vi "test6-Interrupt_Queue.vi"(8 "error in (no error)":errorcluster, 11 "TestCase in":refnum<class "testcase-CSMGlobalLog.lvclass">) -> (0 "error out":errorcluster, 3 "TestCase out":refnum<class "testcase-CSMGlobalLog.lvclass">)   [LabVIEW 2017, in "testcase-CSMGlobalLog.lvclass"]
uses:
  testcase-CSMGlobalLog.lvclass
  testcase-CSMGlobalLog.lvclass/testcase-CSMGlobalLog.ctl
  05ebe40f-4c18-45b8-8385-0deae4bc461c.vi
  74c550d6-8d72-4fbc-9b84-854ca9ba218d.vi
  f2908a69-50b3-4358-8c93-3e573ca7d2ca.vi
  <vilib>/addons/_JKI Toolkits/VI Tester/TestCase.llb/TestCase.lvclass
  src/user.lib/_NEVSTOP/Communicable State Machine(CSM)/Communicable State Machine.lvlib
  src/user.lib/_NEVSTOP/Communicable State Machine(CSM)/Utility/Periodic String Filter Setting.ctl
  CSM/CSM-Testcase.lvlib
  C:/Program Files (x86)/National Instruments/LabVIEW 2017/vi.lib/addons/_JKI Toolkits/VI Tester/TestCase.llb/TestCase.lvclass
panel:
  out "String cache total":string
  out "LoopCount":i32
  out "String Cache Each Loop":string
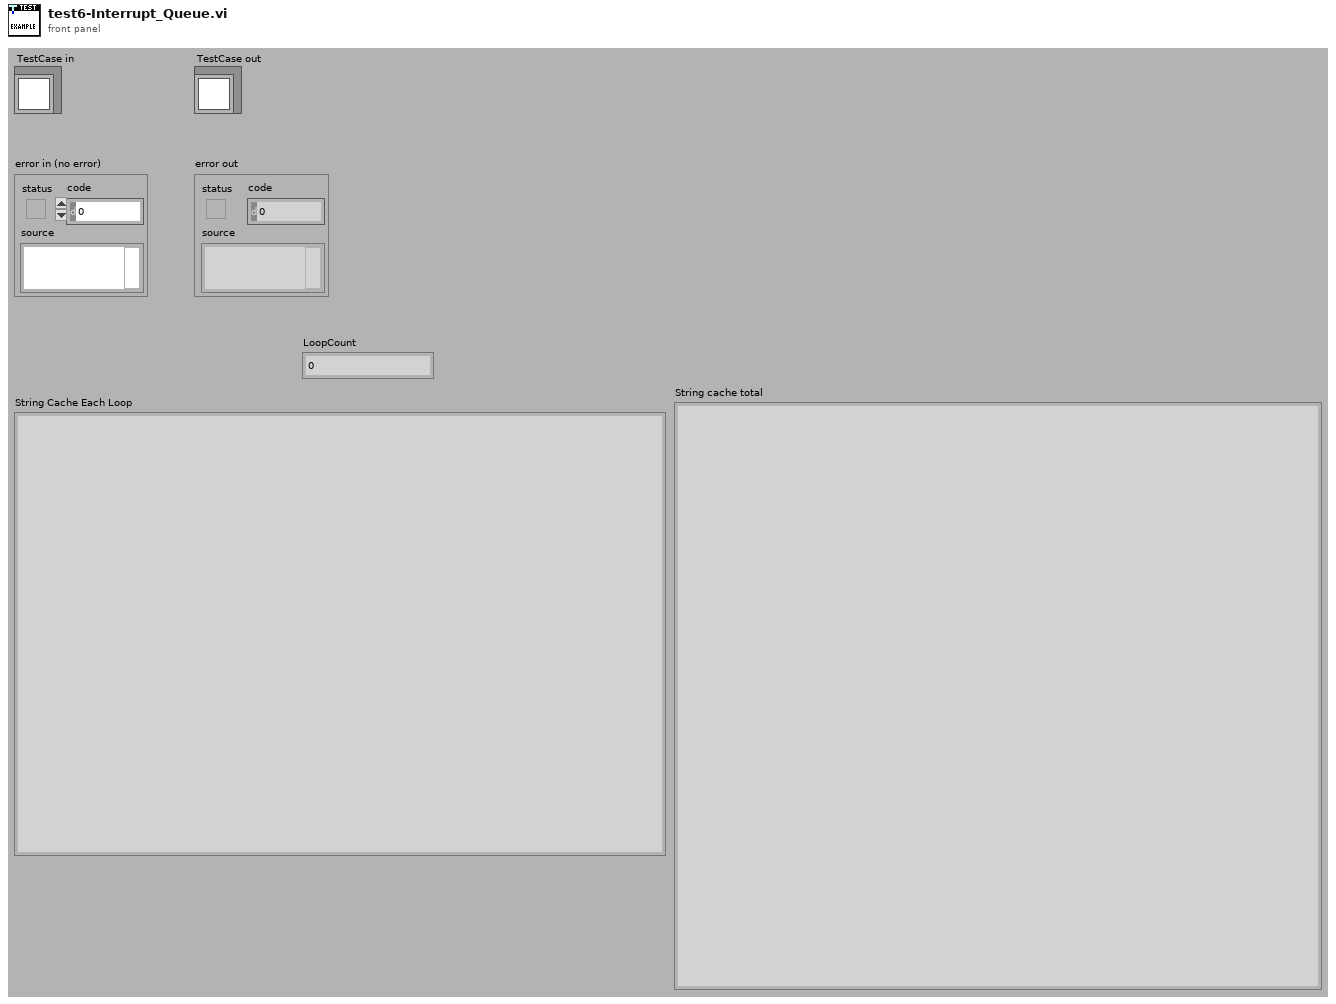
[diagram p1: front panel]
types:
  T1 = typedef "Communicable State Machine.lvlib/Periodic String Filter Setting.ctl" = cluster{"threashold(#/s)":dbl, "Check Peroid(s)":dbl}
  T2 = typedef "Communicable State Machine.lvlib/_CSM_GlobalLog_MSG.ctl" = cluster{"Name (\"\" to Use UUID)":string, "Current State":string, "Arguments":string, "Source Message":T3, "Source Module":string, "Complete(T)/Start(F)":bool, "LogType":T4, "Time Stamp":timestamp}
  T3 = typedef "Communicable State Machine.lvlib/_CSM_Response Source Message.ctl" = cluster{"‘State":string, "’Arguments":string, "’Error":errorcluster}
  T4 = typedef "Communicable State Machine.lvlib/_CSM_GlobalLog_MSG_TYPE.ctl" = enum16{"User Log", "State Change", "Status", "Interrupt", "Register", "Unregister", "Error Log", "Module Created", "Module Destroyed", "Async Message", "No-Rep Async Message", "Sync Message"}
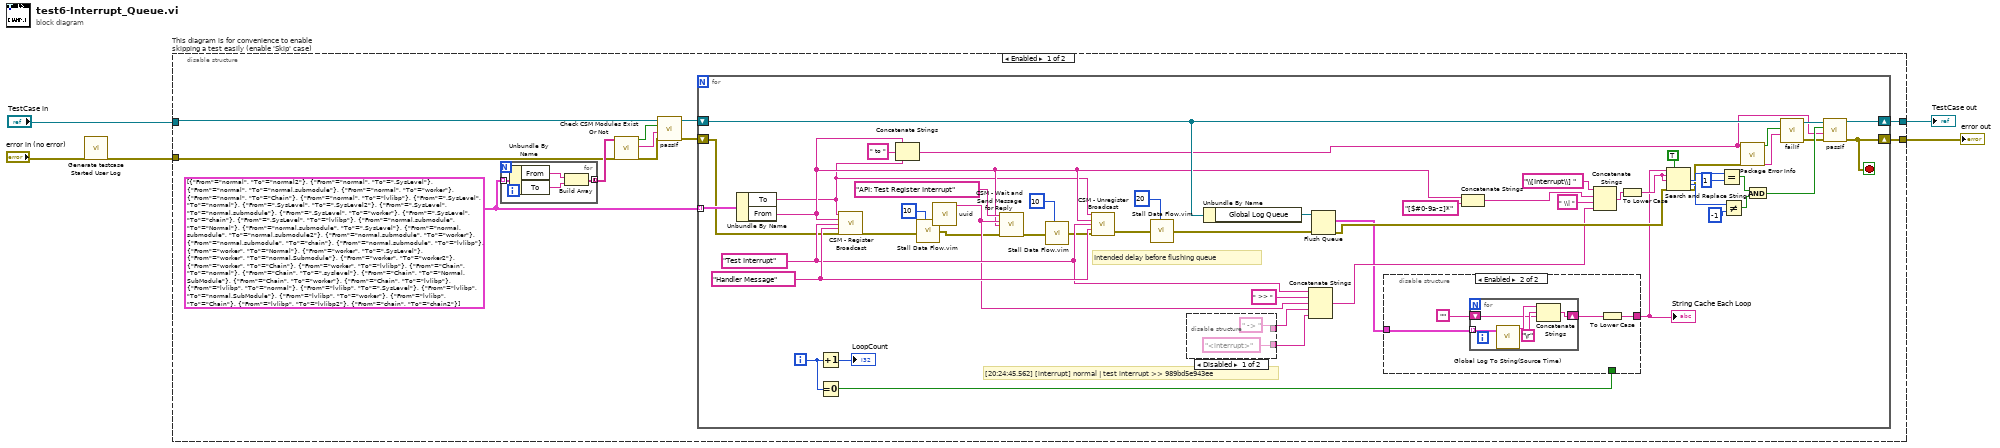
[diagram p0: block diagram]
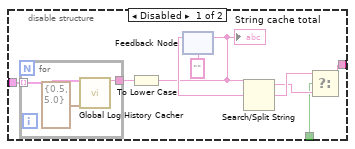
[diagram p3: hidden frame]
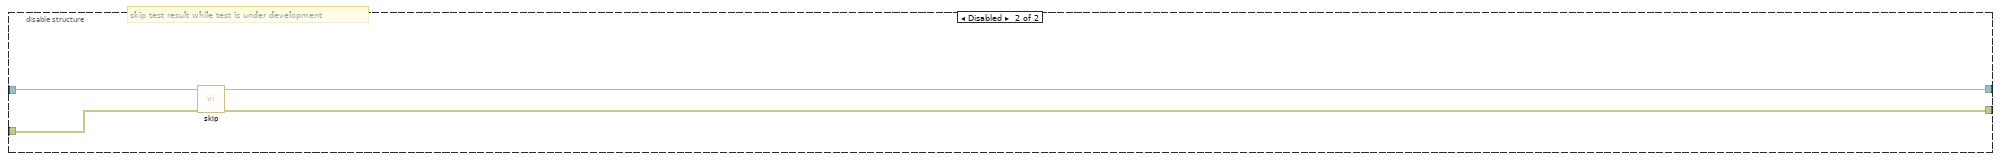
[diagram p4: hidden frame]
diagram:
  n1 = call "Generate testcase Started User Log.vi"("Error In"="error in (no error)") -> ("error out"=w1:errorcluster)  [unwired: 10 in]
  n2 = disable-structure "This diagram is for convenience to enable skipping a test easily (enable 'Skip' case)" shown="Enabled" {
    disable-tunnel: "TestCase in" -> [w9 w99]
    disable-tunnel: [w15 w97] -> w2
    disable-tunnel: [w16 w98] -> w4
    disable-tunnel: w1 -> [w6 w96]
    frame Enabled {
      w10 = cluster{"From":string, "To":string}[] [{"From"="normal", "To"="normal2"}, {"From"="normal", "To"=".SysLevel"}, {"From"="normal", "To"="normal.submodule"}, {"From"="normal", "To"="worker"}, {"From"="normal", "To"="Chain"}, {"From"="normal", "To"="lvlibp"}, {"From"=".SysLevel", "To"="normal"}, {"From"=".SysLevel", "To"=".SysLevel2"}, {"From"=".SysLevel", "To"="normal.submodule"}, {"From"=".SysLevel", "To"="worker"}, {"From"=".SysLevel", "To"="chain"}, {"From"=".SysLevel", "To"="lvlibp"}, {"From"="normal.submodule", "To"="Normal"}, {"From"="normal.submodule", "To"=".SysLevel"}, {"From"="normal.submodule", "To"="normal.submodule2"}, {"From"="normal.submodule", "To"="worker"}, {"From"="normal.submodule", "To"="chain"}, {"From"="normal.submodule", "To"="lvlibp"}, {"From"="worker", "To"="Normal"}, {"From"="worker", "To"=".SysLevel"}, {"From"="worker", "To"="normal.Submodule"}, {"From"="worker", "To"="worker2"}, {"From"="worker", "To"="Chain"}, {"From"="worker", "To"="lvlibp"}, {"From"="Chain", "To"="normal"}, {"From"="Chain", "To"=".syslevel"}, {"From"="Chain", "To"="Normal.SubModule"}, {"From"="Chain", "To"="worker"}, {"From"="Chain", "To"="lvlibp"}, {"From"="lvlibp", "To"="normal"}, {"From"="lvlibp", "To"=".SysLevel"}, {"From"="lvlibp", "To"="normal.SubModule"}, {"From"="lvlibp", "To"="worker"}, {"From"="lvlibp", "To"="Chain"}, {"From"="lvlibp", "To"="lvlibp2"}, {"From"="chain", "To"="chain2"}]
      n3 = for {
        tunnel: w10 -> [w20] mode=indexing
        tunnel: [w17] -> w13 mode=concatenating
        n4 = Unbundle By Name(w20) -> ("From"=w19:string, "To"=w18:string)
        n5 = Build Array(w19, w18) -> (w17:string[])
      }
      n6 = call "Check CSM Modules Exist Or Not.vi"("error in"=w6, "CSM names in"=w13) -> ("error out"=w11:errorcluster, "Debug string"=w12:string, "All Modules Exist?"=w14:bool)  [unwired: 7 in]
      n7 = call-dynamic "passIf.vi"("error in (no error)"=w11, "message (\"\")"=w12, "pass"=w14, "TestCase in"=w9) -> ("error out"=w7:errorcluster, "TestCase out"=w8:refnum<class "testcase-CSMGlobalLog.lvclass">)  [unwired: 6 in]
      n8 = for {
        tunnel: w10 -> [w60] mode=indexing
        shift-right: [w46] -> w16
        shift-left: w7 -> [w37]
        shift-right: [w72] -> w15
        shift-left: w8 -> [w34]
        i -> [w39]
        stop <- w46 stop-if-true
        w59 = "Handler Message" ("API (If \"\", Same as Trigger)")
        w54 = "Test Interrupt" ("Trigger")
        # "[20:24:45.562] [interrupt] normal | test interrupt >> 989bd5e943ee"
        # "Intended delay before flushing queue"
        n9 = Unbundle By Name(w60) -> ("To"=w28:string, "From"=w29:string)
        n10 = Equal To 0?(x=w39) -> (x = 0?=w38:bool)
        n11 = Increment(x=w39) -> (x+1=→"LoopCount":i32)
        n12 = call "CSM - Register Broadcast.vi"("CSM Name(Empty for Broadcast Event)"=w28, "Source CSM Name (* as Default)"=w29, "Trigger"=w54, "API (If \"\", Same as Trigger)"=w59, "Error In"=w37) -> ("error out"=w22:errorcluster)  [unwired: 9 in, 1 out]
        n13 = Concatenate Strings(w29, " to " ("string"), w28) -> (w27:string)
        n14 = call "Stall Data Flow.vim"("value in"=w22, "milliseconds to wait"=u32 10 ("millisecond timer value")) -> ("value out"=w21:errorcluster)  [unwired: 1 out]
        n15 = call "uuid.vi"() -> ("UUID"=w52:string)  [unwired: 11 in]
        n16 = call "CSM - Wait and Send Message for Reply.vi"("State"="API: Test Register Interrupt", "Arguments (\"\")"=w52, "Target Module"=w29, "Error In (No Error)"=w21) -> ("error out"=w25:errorcluster)  [unwired: 8 in, 3 out]
        n17 = call "Stall Data Flow.vim"("value in"=w25, "milliseconds to wait"=u32 10 ("millisecond timer value")) -> ("value out"=w24:errorcluster)  [unwired: 1 out]
        n18 = call "CSM - Unregister Broadcast.vi"("CSM Name(Empty for Broadcast Event)"=w28, "Source CSM Name (* as Default)"=w29, "Trigger"=w54, "API (\"*\" as Default)"=w59, "Error In"=w24) -> ("error out"=w44:errorcluster)  [unwired: 9 in, 1 out]
        n19 = call "Stall Data Flow.vim"("value in"=w44, "milliseconds to wait"=u32 20 ("millisecond timer value")) -> ("value out"=w43:errorcluster)  [unwired: 1 out]
        n20 = disable-structure shown="Disabled" {
          disable-tunnel: [" -> " ("string") _] -> w51
          disable-tunnel: ["<interrupt>" ("search string") _] -> w49
          frame Disabled {
          }
          frame Enabled {
          }
        }
        n21 = Unbundle By Name(w34) -> ("Global Log Queue"=w71:refnum<queue>)
        n22 = Concatenate Strings(w54, " >> " ("string"), w52, w51, w49) -> (w50:string)
        n23 = Flush Queue(queue=w71, error in (no error)=w43) -> (remaining elements=w40:T2[], error out=w62:errorcluster)  [unwired: 1 out]
        n24 = disable-structure shown="Enabled" {
          disable-tunnel: [w77 w87] -> w41
          disable-tunnel: w38 -> [w76 _]
          disable-tunnel: w40 -> [w75 w89]
          frame Disabled {
            n25 = for {
              tunnel: w75 -> [w86] mode=indexing
              tunnel: [w85] -> w83
              n26 = call "Global Log History Cacher.vi"("Global Log Data"=w86, "Settings"=T1 {"threashold(#/s)"=0.5, "Check Peroid(s)"=5.0}) -> ("String Cache"=w85:string)  [unwired: 13 in]
            }
            n27 = To Lower Case(string=w83) -> (all lower case string=w78:string)
            "String cache total" <- w78
            n28 = feedback #1("") -> (w82:string)
            n29 = feedback-in #1(w78) -> ()
            n30 = Search/Split String(string=w78, search string/char (-)=w82) -> (substring before match=w79:string, match + rest of string=w80:string)  [unwired: 1 in, 1 out]
            n31 = Select(t=w80, s=w76, f=w79) -> (s? t:f=w77:string)
          }
          frame Enabled {
            n32 = for {
              tunnel: w89 -> [w95] mode=indexing
              shift-right: [w91] -> w88
              shift-left: "" -> [w92]
              n33 = call "Global Log To String(Source Time).vi"("Log"=w95) -> ("Log String"=w94:string)  [unwired: 9 in]
              n34 = Concatenate Strings(w94, "\r", w92) -> (w91:string)
            }
            n35 = To Lower Case(string=w88) -> (all lower case string=w87:string)
          }
        }
        "String Cache Each Loop" <- w41
        n36 = Concatenate Strings(w29, "[$#0-9a-z]*" ("string")) -> (w47:string)
        n37 = Concatenate Strings("\\[Interrupt\\] " ("regular expression"), w47, " \\| " ("string"), w50) -> (w56:string)
        n38 = To Lower Case(string=w56) -> (all lower case string=w68:string)
        n39 = Search and Replace String(replace all?=TRUE ("replace all? (F)"), input string=w41, search string=w68, replace string=w68, error in=w62) -> (number of replacements=w67:i32, offset past replacement=w66:i32, error out=w31:errorcluster)  [unwired: 3 in, 1 out]
        n40 = Equal?(x=w67, y=1) -> (x = y?=w64:bool)
        n41 = Not Equal?(x=w66, y=-1) -> (x != y?=w63:bool)
        n42 = call "Package Error Info.vi"("error in"=w31, "String in"=w27) -> ("packed error info out"=w36:string, "error status"=w35:bool)  [unwired: 8 in]
        n43 = And(x=w64, y=w63) -> (x .and. y?=w45:bool)
        n44 = call-dynamic "failIf.vi"("message (\"\")"=w36, "fail"=w35, "TestCase in"=w34) -> ("error out"=w32:errorcluster, "TestCase out"=w33:refnum<class "testcase-CSMGlobalLog.lvclass">)  [unwired: 7 in]
        n45 = call-dynamic "passIf.vi"("error in (no error)"=w32, "message (\"\")"=w27, "pass"=w45, "TestCase in"=w33) -> ("error out"=w46:errorcluster, "TestCase out"=w72:refnum<class "testcase-CSMGlobalLog.lvclass">)  [unwired: 6 in]
      }
    }
    frame Disabled {
      # "skip test result while test is under development"
      n46 = call <vilib>:"skip.vi"("error in (no error)"=w96, "TestCase in"=w99) -> ("error out"=w98:errorcluster, "TestCase out"=w97:refnum<class "testcase-CSMGlobalLog.lvclass">)  [unwired: 8 in]
    }
  }
  "error out" <- w4
  "TestCase out" <- w2
